vi "Determine Clicked Array Element Index - Determine Index Values (1D or 2D Array).vi"(9 "Array Property.Index Values":u32[](array[numeric]), 11 "Array Property.Number of Rows":u32) -> (0 "Index Values (1D or 2D Array)":u32[](array[numeric]))   [LabVIEW 2015]
doc: "Determine Clicked Array Element Index - Determine Index Values (1D or 2D Array).vi\n\nDescription:\nThis VI determines the index values for 1D or 2D arrays. If the array is a 1D array, this VI outputs the correct index values whether the array is displayed horizontally or vertically.\n\nInputs:\nArray Property.Index Values - Index values returned from the array property node.\n\nArray Property.Number of Rows - Number of rows returned from the array property node.\n\nOutputs:\nIndex Values (1D or 2D Array) - The index values for a 1D or 2D array.\n\nDeveloped By:\nMark.ridgley\nMark.Ridgley_LabVIEW.Developer@comcast.net"
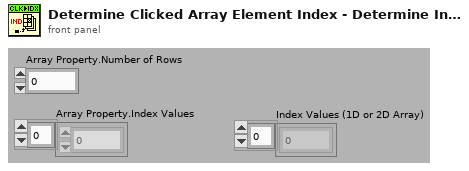
[diagram p1: front panel]
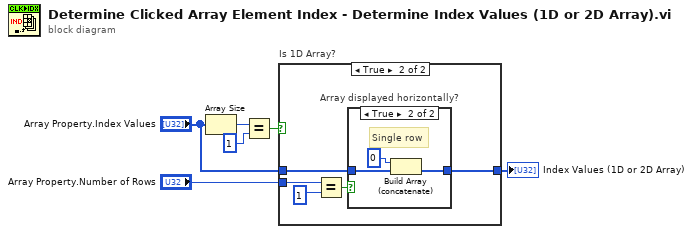
[diagram p0: block diagram]
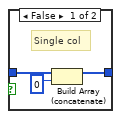
[diagram p3: hidden frame]
diagram:
  n1 = Array Size(array="Array Property.Index Values") -> (size(s)=w2:i32)
  n2 = Equal?(x=w2, y=1) -> (x = y?=w3:bool)
  n3 = case "Is 1D Array?" shown="True" w3 {
    tunnel: "Array Property.Number of Rows" -> [_ w11]
    tunnel: [w7 w9] -> w5
    tunnel: "Array Property.Index Values" -> [w7 w8]
    frame False {
    }
    frame True {
      n4 = Equal?(x=w11, y=u32 1) -> (x = y?=w12:bool)
      n5 = case "Array displayed horizontally?" shown="True" w12 {
        tunnel: w8 -> [w15 w18]
        tunnel: [w14 w17] -> w9
        frame False {
          # "Single col"
          n6 = Build Array (concatenate)(w15, u32 0) -> (w14:u32[])
        }
        frame True {
          # "Single row"
          n7 = Build Array (concatenate)(u32 0, w18) -> (w17:u32[])
        }
      }
    }
  }
  "Index Values (1D or 2D Array)" <- w5
